vi "Timestamp to us.vi"(4 "Timestamp":dbl format="%<%H:%M:%S%3u\n%m/%d/%Y>T") -> (7 "Timestamp us":i64)   [LabVIEW 2020, in "Vecto.lvlib"]
uses:
  Vecto.lvlib
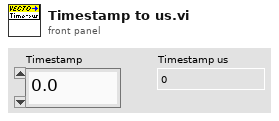
[diagram p1: front panel]
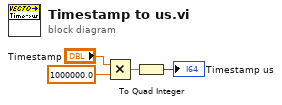
[diagram p0: block diagram]
diagram:
  n1 = Multiply(x="Timestamp", y=1000000.0) -> (x*y=w2:dbl)
  n2 = To Quad Integer(1:w2) -> (0:→"Timestamp us":i64)
